vi "Measurement Visualization.vi"(8 "error in (no error)":errorcluster, 11 "SCADA in":refnum<class "SCADA.lvclass">) -> (0 "error out":errorcluster, 3 "SCADA out":refnum<class "SCADA.lvclass">)   [LabVIEW 2015, in "SCADA Core.lvlib" / "SCADA.lvclass"]
doc: "This takes a comma-delimited list of IED Names and Measurement Names and returns the measurements as a double array flattened to a string."
uses:
  SCADA.lvclass
  SCADA Abstract Messages/IED Measurement Status Msg/IED Measurement Status.ctl
  <vilib>/ActorFramework/Actor/Actor.lvclass/Actor.ctl
  SCADA.lvclass/SCADA.ctl
  <vilib>/NI/Tools/Keyed Array/Map String.vi
  <vilib>/NI/Tools/String/Get Case Matching.vi
  <vilib>/NI/Tools/Keyed Array/Tools_KeyedArray.lvlib
  <vilib>/ActorFramework/Actor/Actor.lvclass
  SCADA Abstract Messages/IED Measurement Status Msg/IED Measurement Status Msg.lvclass
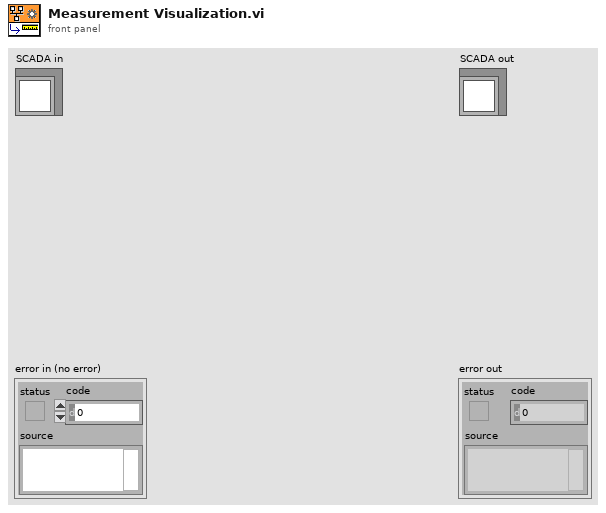
[diagram p1: front panel]
types:
  T1 = typedef "SCADA Core.lvlib/IED Measurement Status Msg.lvclass/IED Measurement Status.ctl" = enum16{"Single Success", "Single Failure", "Multiple Success", "Multiple Failure"}
  T2 = typedef "Tools_KeyedArray.lvlib/KeyedArray.ctl" = cluster{"keys":string[], "values":string[]}
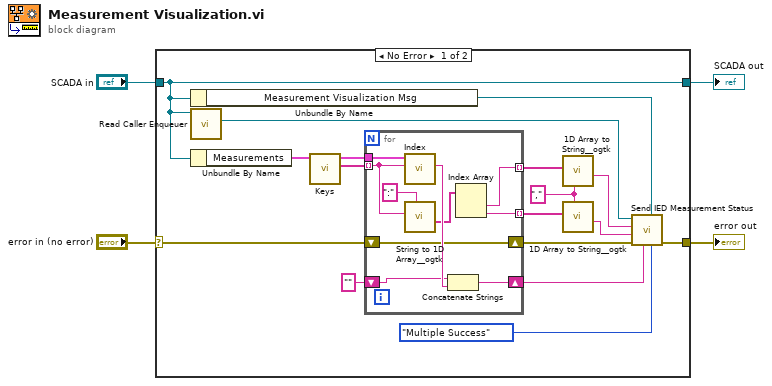
[diagram p0: block diagram]
diagram:
  n1 = case shown="No Error" "error in (no error)" {
    selector: "error in (no error)" -> [w21 w33]
    tunnel: [w16 w33] -> w3
    tunnel: [w20 w32] -> w1
    tunnel: "SCADA in" -> [w20 w32]
    frame No Error {
      w12 = "," ("delimiter (Tab)")
      n2 = Unbundle By Name(w20) -> ("Measurement Visualization Msg"=w19:refnum<class "IED Measurement Status Msg.lvclass">)
      n3 = call <vilib>:"Read Caller Enqueuer.vi"("Actor"=w20) -> ("Caller Enqueuer"=w18:refnum<class "Message Enqueuer.lvclass">)  [unwired: 10 in]
      n4 = Unbundle By Name(w20) -> ("Measurements"=w8:T2)
      n5 = call <vilib>:"Keys.vi"("array in"=w8) -> ("keys"=w7:string[], "duplicate array"=w6:T2)  [unwired: 5 in]
      n6 = for {
        tunnel: [w24] -> w15 mode=indexing
        tunnel: [w23] -> w13 mode=indexing
        shift-right: [w30] -> w17
        shift-left: w21 -> [w30]
        shift-right: [w29] -> w9
        shift-left: "" ("value") -> [w28]
        tunnel: w7 -> [w26] mode=indexing
        tunnel: w6 -> [w22]
        n7 = call <vilib>:"Index.vi"("key"=w26, "array in"=w22) -> ("value"=w31:string)  [unwired: 3 in, 2 out]
        n8 = call <userlib>:"String to 1D Array__ogtk.vi"("delimiter (Tab)"=":" ("string"), "string"=w26) -> ("Array of Strings"=w25:string[])  [unwired: 9 in]
        n9 = Concatenate Strings(w28, w31) -> (w29:string)
        n10 = Index Array(array=w25) -> (element #1=w24:string, element #2=w23:string)  [unwired: 2 in]
      }
      n11 = call <userlib>:"1D Array to String__ogtk.vi"("delimiter (Tab)"=w12, "Array of Strings"=w15) -> ("delimited string"=w14:string)  [unwired: 9 in]
      n12 = call <userlib>:"1D Array to String__ogtk.vi"("delimiter (Tab)"=w12, "Array of Strings"=w13) -> ("delimited string"=w11:string)  [unwired: 9 in]
      n13 = call "Send IED Measurement Status.vi"("Status"=IED_Measurement_Status."Multiple Success", "IED Measurement Msg"=w19, "Value/error"=w9, "error in (no error)"=w17, "Measurement Name"=w11, "IED Name"=w14, "Message Enqueuer in"=w18) -> ("error out"=w16:errorcluster)  [unwired: 3 in, 1 out]
    }
    frame Error {
    }
  }
  "error out" <- w3
  "SCADA out" <- w1
